vi "Close FlexLogger Project.vi"(6 "timeout (ms)":i32=-1, 8 "error in (no error)":errorcluster, 11 "FlexLogger_gRPCAPI in":refnum<class "FlexLogger_gRPC.lvclass">) -> (0 "error out":errorcluster, 2 "timed out?":bool, 3 "FlexLogger_gRPCAPI out":refnum<class "FlexLogger_gRPC.lvclass">)   [LabVIEW 2020, in "FlexLogger_gRPC.lvlib" / "FlexLogger_gRPC.lvclass"]
uses:
  FlexLogger_gRPC.lvclass
  FlexLogger_client/RPC Messages/flexlogger_ProjectIdentifier.ctl
  FlexLogger_client/RPC Messages/flexlogger_ElementIdentifier.ctl
  FlexLogger_gRPC.lvclass/FlexLogger_gRPC.ctl
  FlexLogger_client/FlexLogger_client.lvlib
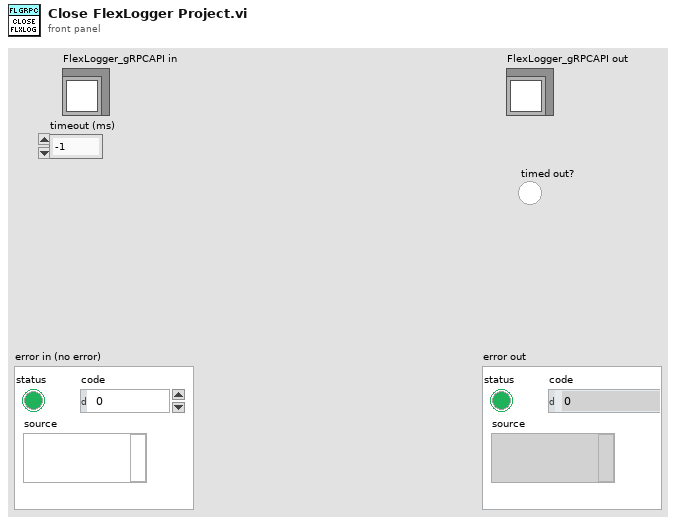
[diagram p1: front panel]
types:
  T1 = typedef "FlexLogger_client.lvlib/flexlogger_ElementIdentifier.ctl" = cluster{"project_id":string, "file_name":string, "element_id":string, "subpart_id":string}
  T2 = typedef "FlexLogger_client.lvlib/flexlogger_ProjectIdentifier.ctl" = cluster{"project_id":string}
  T3 = typedef "grpc-lvsupport-release.lvlib/grpcId.ctl" = u64
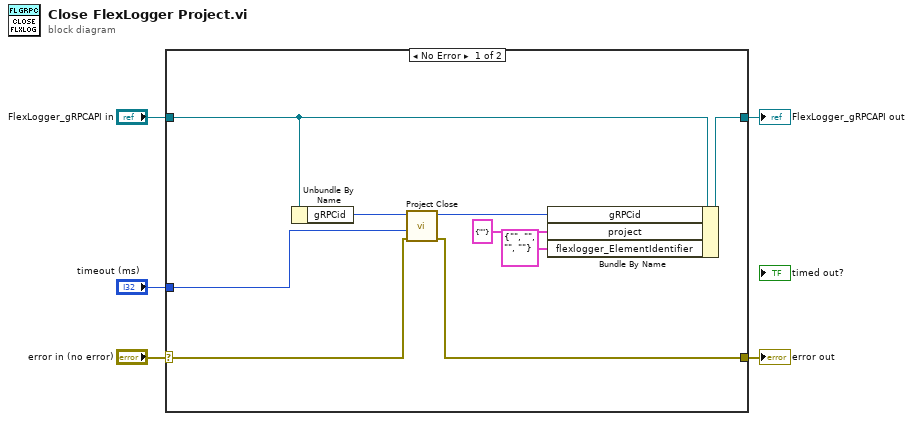
[diagram p0: block diagram]
diagram:
  n1 = case shown="No Error" "error in (no error)" {
    selector: "error in (no error)" -> [w10 w15]
    tunnel: [w9 w15] -> w4
    tunnel: [w13 w16] -> w3
    tunnel: "FlexLogger_gRPCAPI in" -> [w12 w16]
    tunnel: "timeout (ms)" -> [w6 _]
    frame No Error {
      n2 = Unbundle By Name(w12) -> ("gRPCid"=w14:T3)
      n3 = call "Project Close.vi"("error in"=w10, "timeout (ms)"=w6, "gRPC ID"=w14) -> ("error out"=w9:errorcluster, "gRPC ID out"=w11:T3)  [unwired: 6 in, 1 out]
      n4 = Bundle By Name(cluster=w12, "gRPCid"=w11, "project"=T2 {"project_id"=""}, "flexlogger_ElementIdentifier"=T1 {"project_id"="", "file_name"="", "element_id"="", "subpart_id"=""}) -> (w13:refnum<class "FlexLogger_gRPC.lvclass">)
    }
    frame Error {
    }
  }
  "error out" <- w4
  "FlexLogger_gRPCAPI out" <- w3
